vi "Build CHM Help.vi"(8 "error in":errorcluster, 11 "Main Destination Path":path) -> (0 "error out":errorcluster)   [LabVIEW 2020]
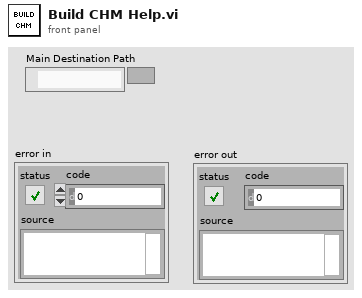
[diagram p1: front panel]
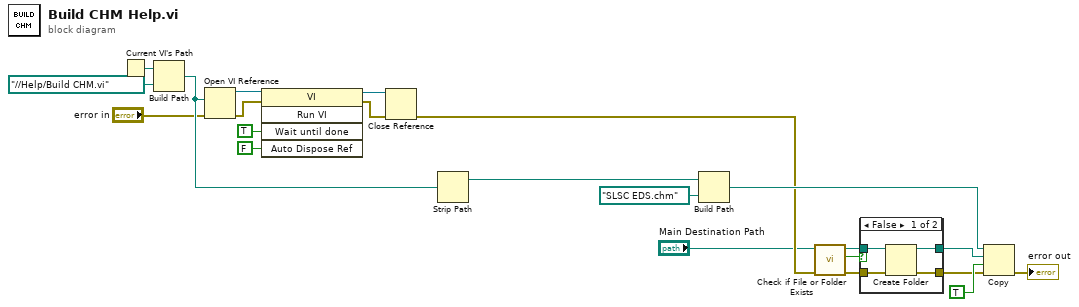
[diagram p0: block diagram]
diagram:
  n1 = Current VI's Path() -> (path=w2:path)
  n2 = Build Path(base path=w2, name or relative path=path "../../Help/Build CHM.vi") -> (appended path=w10:path)
  n3 = Open VI Reference(vi path=w10, error in (no error)="error in") -> (vi reference=w4:refnum<vi>, error out=w5:errorcluster)  [unwired: 4 in]
  n4 = invoke class="VI" method="Run VI"(reference=w4, error in=w5, "Wait until done"=TRUE ("Wait Until Done"), "Auto Dispose Ref"=FALSE ("Auto Dispose Reference")) -> (reference out=w8:refnum<vi>, error out=w9:errorcluster)  [unwired: 1 in, 3 out]
  n5 = Close Reference(reference=w8, error in (no error)=w9) -> (error out=w12:errorcluster)
  n6 = Strip Path(path=w10) -> (stripped path=w21:path)  [unwired: 1 out]
  n7 = Build Path(base path=w21, name or relative path=path "SLSC EDS.chm") -> (appended path=w19:path)
  n8 = call <vilib>:"Check if File or Folder Exists.vi"("error in (no error)"=w12, "path"="Main Destination Path") -> ("error out"=w15:errorcluster, "file or folder exists?"=w13:bool, "dup path"=w14:path)  [unwired: 7 in]
  n9 = case shown="False" w13 {
    tunnel: w14 -> [w25 w28]
    tunnel: w15 -> [w26 w27]
    tunnel: [w24 w28] -> w17
    tunnel: [w23 w27] -> w16
    frame False {
      n10 = Create Folder(path (use dialog)=w25, error in=w26) -> (created path=w24:path, error out=w23:errorcluster)  [unwired: 1 in, 1 out]
    }
    frame True {
    }
  }
  n11 = Copy(8:w16, 9:TRUE ("overwrite (F)"), 10:w17, 11:w19) -> (0:→"error out":errorcluster)  [unwired: 1 in, 2 out]
